vi "FGV.vi"(8 "error in (no error)":errorcluster) -> (0 "error out":errorcluster, 2 "Valve ON":bool)   [LabVIEW 2010]
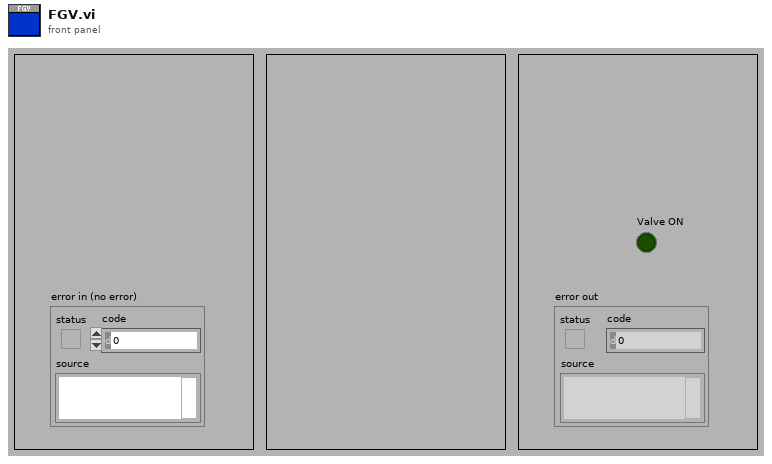
[diagram p1: front panel]
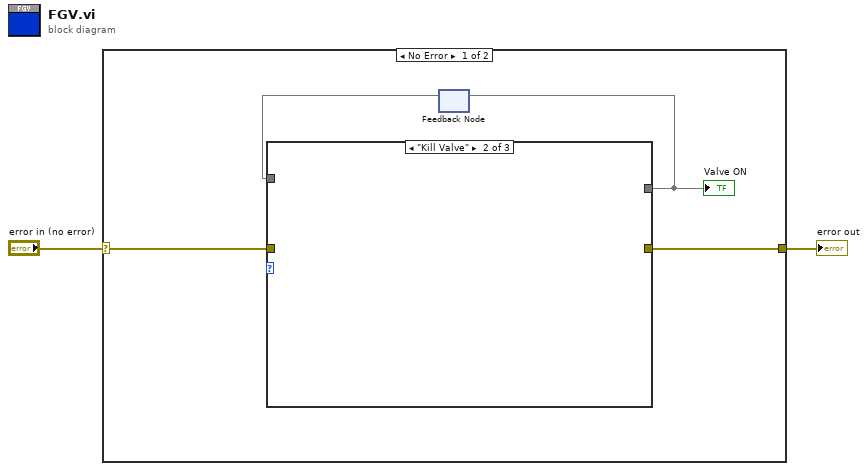
[diagram p0: block diagram]
diagram:
  n1 = case shown="No Error" "error in (no error)" {
    selector: "error in (no error)" -> [w6 w15]
    tunnel: [w5 w15] -> w1
    frame No Error {
      n2 = feedback #1() -> (w3)  [unwired: 1 in]
      n3 = case shown="\"Kill Valve\"" {
        selector: _ -> [_ _ _]
        tunnel: w6 -> [w9 w12 w13]
        tunnel: [w8 w11 w13] -> w5
        tunnel: [w7 w10 w14] -> w4
        tunnel: w3 -> [_ _ w14]
        frame "Run Valve" {
        }
        frame "Kill Valve" {
        }
        frame "Pass" {
        }
      }
      "Valve ON" <- w4
      n4 = feedback-in #1(w4) -> ()
    }
    frame Error {
    }
  }
  "error out" <- w1
